vi "update eol result.vi"(7 "Eol数据":string[](array[string]), 11 "Station Index":i32) -> ()   [LabVIEW 2018]
panel:
  in  "error in (no error)":errorcluster
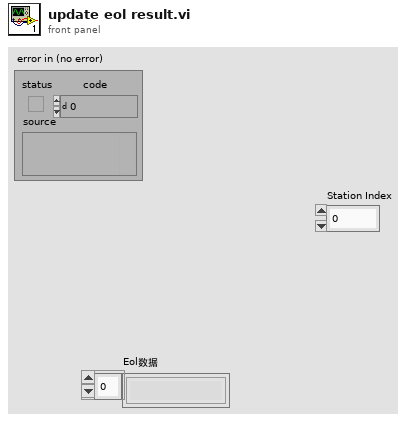
[diagram p1: front panel]
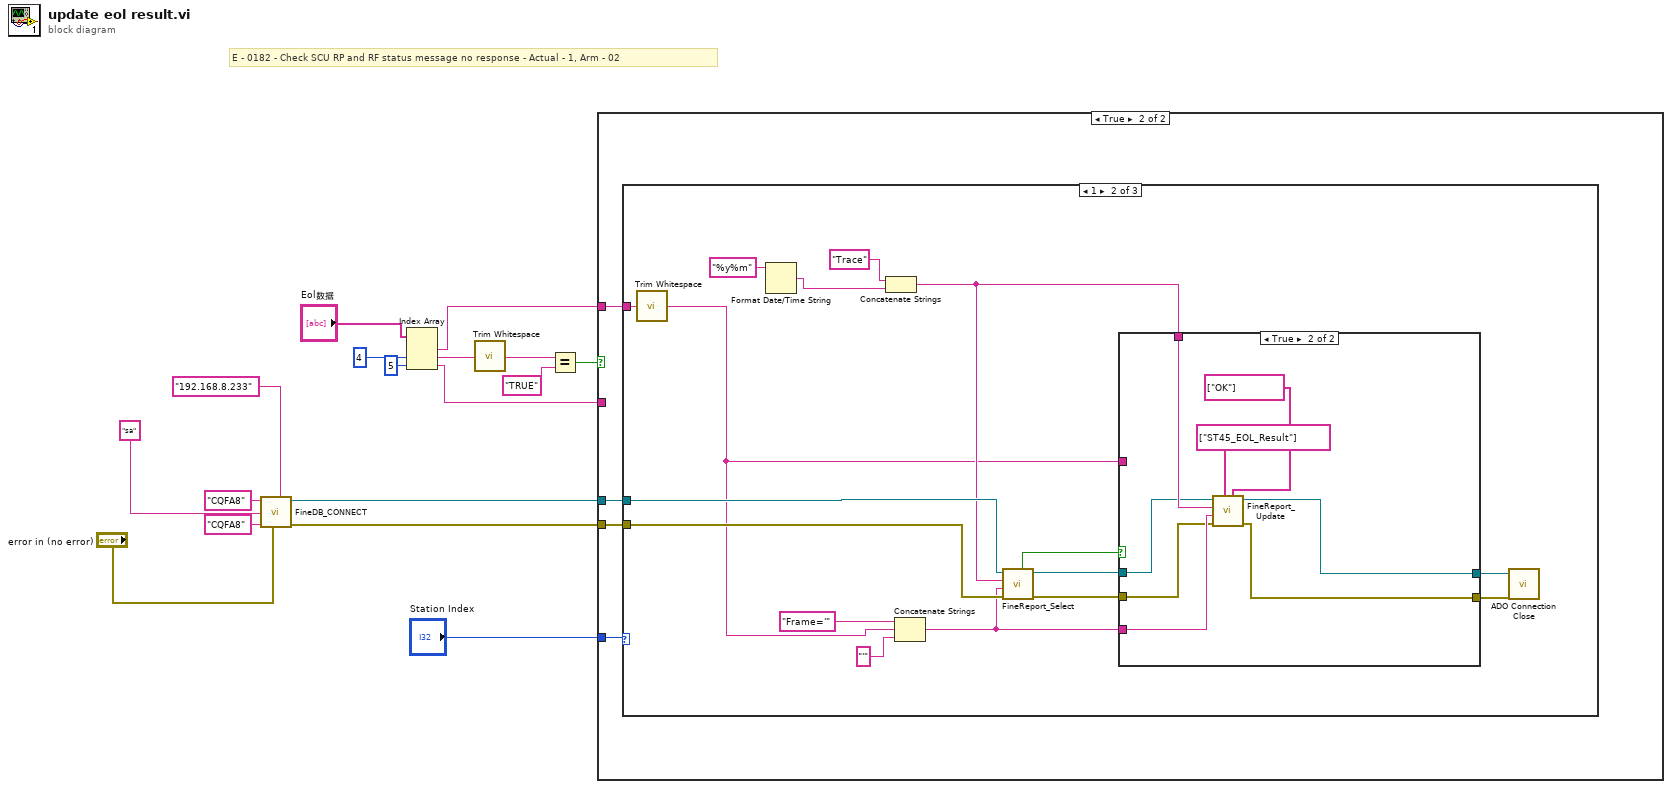
[diagram p0: block diagram]
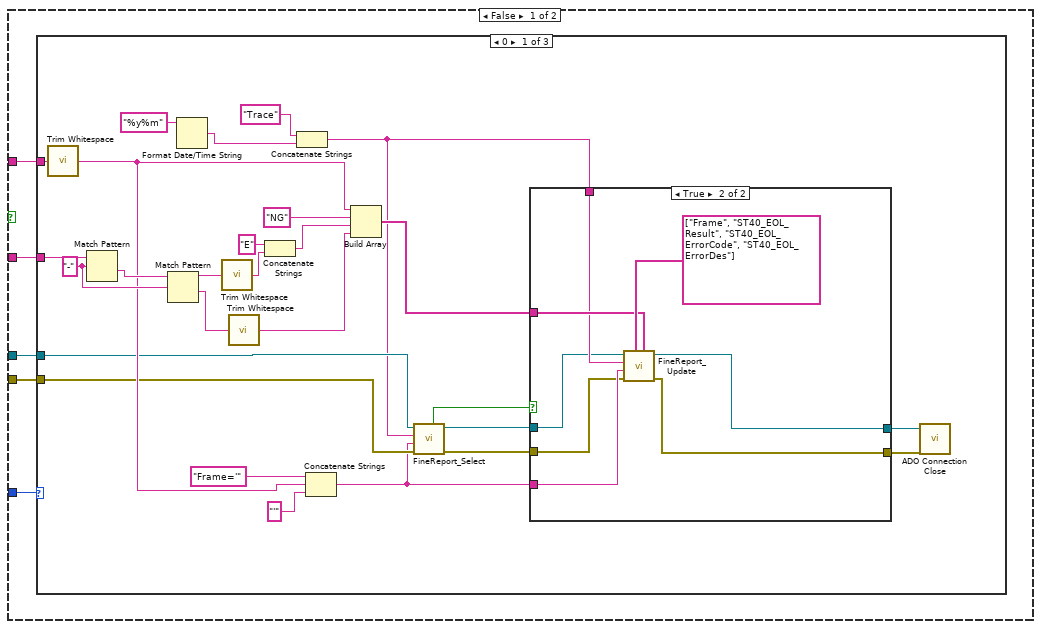
[diagram p2: hidden frame]
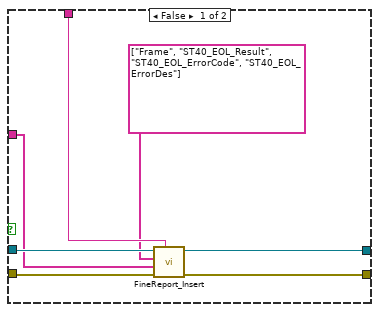
[diagram p3: hidden frame]
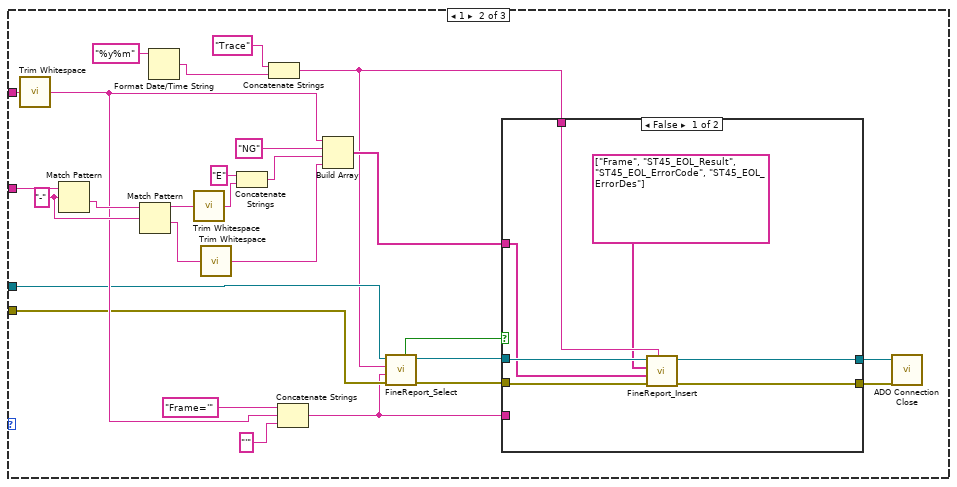
[diagram p4: hidden frame]
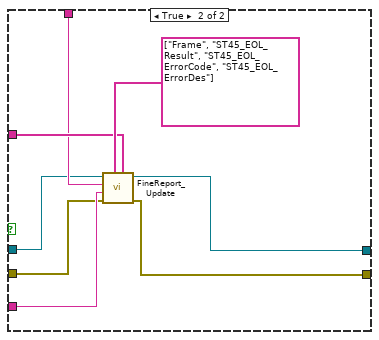
[diagram p5: hidden frame]
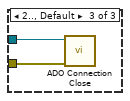
[diagram p6: hidden frame]
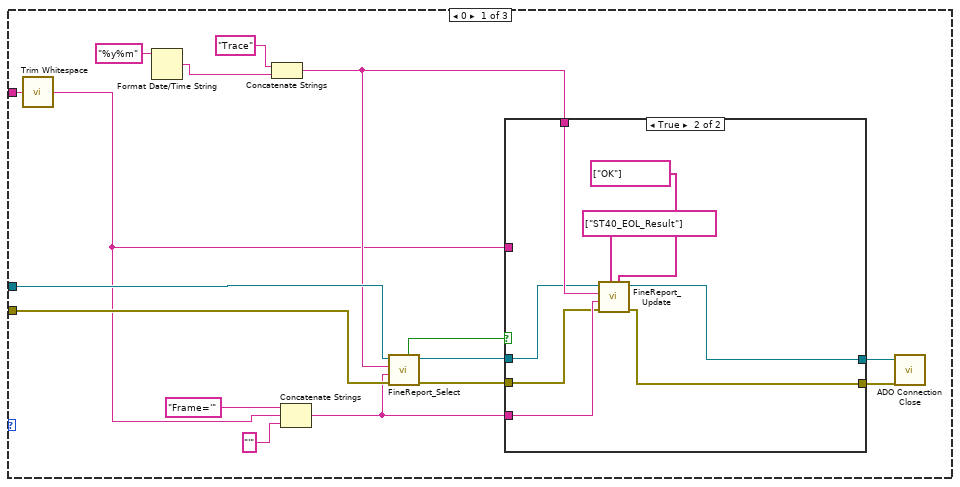
[diagram p7: hidden frame]
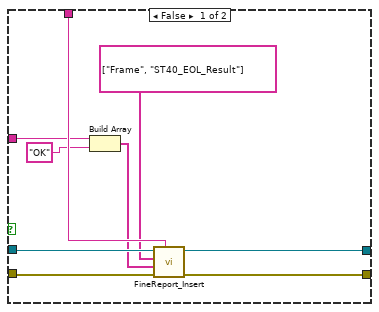
[diagram p8: hidden frame]
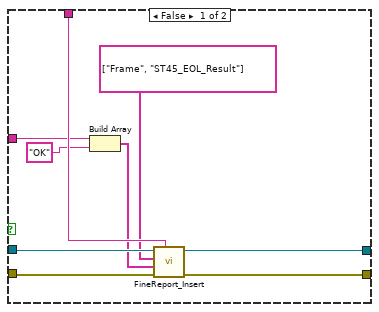
[diagram p9: hidden frame]
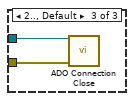
[diagram p10: hidden frame]
diagram:
  # "E - 0182 - Check SCU RP and RF status message no response - Actual - 1, Arm - 02"
  n1 = call "FineDB_CONNECT.vi"("SQL Server_Hostname"="192.168.8.233", "error in (no error)"="error in (no error)", "password"="CQFA8", "account"="sa", "DB_name"="CQFA8") -> ("error out"=w4:errorcluster, "ADODB._Connection Out"=w5:refnum<k7>)  [unwired: 5 in]
  n2 = Index Array(array="Eol数据", index #2=4 ("索引"), index #3=5 ("索引")) -> (element #1=w3:string, element #2=w9:string, element #3=w2:string)  [unwired: 1 in]
  n3 = call <vilib>:"Trim Whitespace.vi"("string"=w9) -> ("trimmed string"=w8:string)  [unwired: 1 in]
  n4 = Equal?(x=w8, y="TRUE") -> (x = y?=w6:bool)
  n5 = case shown="True" w6 {
    tunnel: w5 -> [w20 w111]
    tunnel: w4 -> [w19 w110]
    tunnel: w3 -> [w21 w112]
    tunnel: w2 -> [w22 _]
    tunnel: "Station Index" -> [w18 w109]
    frame False {
      n6 = case shown="0" w18 {
        tunnel: w22 -> [w49 w91 _]
        tunnel: w21 -> [w42 w84 _]
        tunnel: w20 -> [w31 w73 w108]
        tunnel: w19 -> [w30 w72 w107]
        frame 0 {
          w48 = "-" ("正则表达式")
          n7 = call <vilib>:"Trim Whitespace.vi"("string"=w42) -> ("trimmed string"=w34:string)  [unwired: 1 in]
          n8 = Match Pattern(string=w49, regular expression=w48) -> (after substring=w47:string)  [unwired: 1 in, 3 out]
          n9 = Match Pattern(string=w47, regular expression=w48) -> (before substring=w46:string, after substring=w43:string)  [unwired: 1 in, 2 out]
          n10 = Format Date/Time String(time format string (%c)="%y%m" ("时间格式字符串(%c)")) -> (date/time string=w39:string)  [unwired: 2 in]
          n11 = call <vilib>:"Trim Whitespace.vi"("string"=w46) -> ("trimmed string"=w45:string)  [unwired: 1 in]
          n12 = call <vilib>:"Trim Whitespace.vi"("string"=w43) -> ("trimmed string"=w37:string)  [unwired: 1 in]
          n13 = Concatenate Strings("E" ("字符串"), w45) -> (w38:string)
          n14 = Concatenate Strings("Trace", w39) -> (w29:string)
          n15 = Concatenate Strings("Frame='", w34, "'" ("字符串")) -> (w28:string)
          n16 = Build Array(w34, "NG" ("元素"), w38, w37) -> (w32:string[])
          n17 = call "FineReport_Select.vi"("error in (no error)"=w30, "SelectWhere"=w28, "SelectTableName"=w29, "ADODB._Connection in"=w31) -> ("error out"=w25:errorcluster, "ADODB._Connection Out"=w26:refnum<k7>, "有数据"=w27:bool)  [unwired: 3 in, 2 out]
          n18 = case shown="True" w27 {
            tunnel: w32 -> [w52 w63]
            tunnel: w29 -> [w54 w62]
            tunnel: w28 -> [_ w61]
            tunnel: w26 -> [w56 w60]
            tunnel: w25 -> [w55 w59]
            tunnel: [w51 w58] -> w23
            tunnel: [w50 w57] -> w24
            frame False {
              n19 = call "FineReport_Insert.vi"("InsertTableName"=w54, "error in"=w55, "InsertValue(array)"=w52, "InsertColumn(array)"=string[] ["Frame", "ST40_EOL_Result", "ST40_EOL_ErrorCode", "ST40_EOL_ErrorDes"], "ADODB._Connection in"=w56) -> ("error out"=w50:errorcluster, "ADODB._Connection Out"=w51:refnum<k7>)  [unwired: 5 in]
            }
            frame True {
              n20 = call "FineReport_Update.vi"("UpdataValue(array)"=w63, "UpdataColumn(array)"=string[] ["Frame", "ST40_EOL_Result", "ST40_EOL_ErrorCode", "ST40_EOL_ErrorDes"], "error in (no error)"=w59, "UpdataWhere"=w61, "UpdataTableName"=w62, "ADODB._Connection in"=w60) -> ("error out"=w57:errorcluster, "ADODB._Connection Out"=w58:refnum<k7>)  [unwired: 2 in]
            }
          }
          n21 = call <userlib>:"ADO Connection Close.vi"("error in (no error)"=w24, "ADODB._Connection In"=w23) -> ()  [unwired: 8 in, 2 out]
        }
        frame 1 {
          w90 = "-" ("正则表达式")
          n22 = call <vilib>:"Trim Whitespace.vi"("string"=w84) -> ("trimmed string"=w76:string)  [unwired: 1 in]
          n23 = Match Pattern(string=w91, regular expression=w90) -> (after substring=w89:string)  [unwired: 1 in, 3 out]
          n24 = Match Pattern(string=w89, regular expression=w90) -> (before substring=w88:string, after substring=w85:string)  [unwired: 1 in, 2 out]
          n25 = Format Date/Time String(time format string (%c)="%y%m" ("时间格式字符串(%c)")) -> (date/time string=w81:string)  [unwired: 2 in]
          n26 = call <vilib>:"Trim Whitespace.vi"("string"=w88) -> ("trimmed string"=w87:string)  [unwired: 1 in]
          n27 = call <vilib>:"Trim Whitespace.vi"("string"=w85) -> ("trimmed string"=w79:string)  [unwired: 1 in]
          n28 = Concatenate Strings("E" ("字符串"), w87) -> (w80:string)
          n29 = Concatenate Strings("Trace", w81) -> (w71:string)
          n30 = Concatenate Strings("Frame='", w76, "'" ("字符串")) -> (w70:string)
          n31 = Build Array(w76, "NG" ("元素"), w80, w79) -> (w74:string[])
          n32 = call "FineReport_Select.vi"("error in (no error)"=w72, "SelectWhere"=w70, "SelectTableName"=w71, "ADODB._Connection in"=w73) -> ("error out"=w67:errorcluster, "ADODB._Connection Out"=w68:refnum<k7>, "有数据"=w69:bool)  [unwired: 3 in, 2 out]
          n33 = case shown="False" w69 {
            tunnel: w74 -> [w94 w105]
            tunnel: w71 -> [w96 w104]
            tunnel: w70 -> [_ w103]
            tunnel: w68 -> [w98 w102]
            tunnel: w67 -> [w97 w101]
            tunnel: [w93 w100] -> w65
            tunnel: [w92 w99] -> w66
            frame False {
              n34 = call "FineReport_Insert.vi"("InsertTableName"=w96, "error in"=w97, "InsertValue(array)"=w94, "InsertColumn(array)"=string[] ["Frame", "ST45_EOL_Result", "ST45_EOL_ErrorCode", "ST45_EOL_ErrorDes"], "ADODB._Connection in"=w98) -> ("error out"=w92:errorcluster, "ADODB._Connection Out"=w93:refnum<k7>)  [unwired: 5 in]
            }
            frame True {
              n35 = call "FineReport_Update.vi"("UpdataValue(array)"=w105, "UpdataColumn(array)"=string[] ["Frame", "ST45_EOL_Result", "ST45_EOL_ErrorCode", "ST45_EOL_ErrorDes"], "error in (no error)"=w101, "UpdataWhere"=w103, "UpdataTableName"=w104, "ADODB._Connection in"=w102) -> ("error out"=w99:errorcluster, "ADODB._Connection Out"=w100:refnum<k7>)  [unwired: 2 in]
            }
          }
          n36 = call <userlib>:"ADO Connection Close.vi"("error in (no error)"=w66, "ADODB._Connection In"=w65) -> ()  [unwired: 8 in, 2 out]
        }
        frame 2.., Default {
          n37 = call <userlib>:"ADO Connection Close.vi"("error in (no error)"=w107, "ADODB._Connection In"=w108) -> ()  [unwired: 8 in, 2 out]
        }
      }
    }
    frame True {
      n38 = case shown="1" w109 {
        tunnel: w112 -> [w128 w161 _]
        tunnel: w111 -> [w122 w155 w180]
        tunnel: w110 -> [w121 w154 w179]
        frame 0 {
          n39 = call <vilib>:"Trim Whitespace.vi"("string"=w128) -> ("trimmed string"=w113:string)  [unwired: 1 in]
          n40 = Format Date/Time String(time format string (%c)="%y%m" ("时间格式字符串(%c)")) -> (date/time string=w125:string)  [unwired: 2 in]
          n41 = Concatenate Strings("Trace", w125) -> (w120:string)
          n42 = Concatenate Strings("Frame='", w113, "'" ("字符串")) -> (w119:string)
          n43 = call "FineReport_Select.vi"("error in (no error)"=w121, "SelectWhere"=w119, "SelectTableName"=w120, "ADODB._Connection in"=w122) -> ("error out"=w116:errorcluster, "ADODB._Connection Out"=w117:refnum<k7>, "有数据"=w118:bool)  [unwired: 3 in, 2 out]
          n44 = case shown="True" w118 {
            tunnel: w120 -> [w135 w144]
            tunnel: w119 -> [_ w143]
            tunnel: w117 -> [w137 w142]
            tunnel: w116 -> [w136 w141]
            tunnel: [w133 w140] -> w114
            tunnel: [w132 w139] -> w115
            tunnel: w113 -> [w131 _]
            frame False {
              n45 = Build Array(w131, "OK") -> (w129:string[])
              n46 = call "FineReport_Insert.vi"("InsertTableName"=w135, "error in"=w136, "InsertValue(array)"=w129, "InsertColumn(array)"=string[] ["Frame", "ST40_EOL_Result"], "ADODB._Connection in"=w137) -> ("error out"=w132:errorcluster, "ADODB._Connection Out"=w133:refnum<k7>)  [unwired: 5 in]
            }
            frame True {
              n47 = call "FineReport_Update.vi"("UpdataValue(array)"=string[] ["OK"], "UpdataColumn(array)"=string[] ["ST40_EOL_Result"], "error in (no error)"=w141, "UpdataWhere"=w143, "UpdataTableName"=w144, "ADODB._Connection in"=w142) -> ("error out"=w139:errorcluster, "ADODB._Connection Out"=w140:refnum<k7>)  [unwired: 2 in]
            }
          }
          n48 = call <userlib>:"ADO Connection Close.vi"("error in (no error)"=w115, "ADODB._Connection In"=w114) -> ()  [unwired: 8 in, 2 out]
        }
        frame 1 {
          n49 = call <vilib>:"Trim Whitespace.vi"("string"=w161) -> ("trimmed string"=w146:string)  [unwired: 1 in]
          n50 = Format Date/Time String(time format string (%c)="%y%m" ("时间格式字符串(%c)")) -> (date/time string=w158:string)  [unwired: 2 in]
          n51 = Concatenate Strings("Trace", w158) -> (w153:string)
          n52 = Concatenate Strings("Frame='", w146, "'" ("字符串")) -> (w152:string)
          n53 = call "FineReport_Select.vi"("error in (no error)"=w154, "SelectWhere"=w152, "SelectTableName"=w153, "ADODB._Connection in"=w155) -> ("error out"=w149:errorcluster, "ADODB._Connection Out"=w150:refnum<k7>, "有数据"=w151:bool)  [unwired: 3 in, 2 out]
          n54 = case shown="True" w151 {
            tunnel: w153 -> [w168 w177]
            tunnel: w152 -> [_ w176]
            tunnel: w150 -> [w170 w175]
            tunnel: w149 -> [w169 w174]
            tunnel: [w166 w173] -> w147
            tunnel: [w165 w172] -> w148
            tunnel: w146 -> [w164 _]
            frame False {
              n55 = Build Array(w164, "OK") -> (w162:string[])
              n56 = call "FineReport_Insert.vi"("InsertTableName"=w168, "error in"=w169, "InsertValue(array)"=w162, "InsertColumn(array)"=string[] ["Frame", "ST45_EOL_Result"], "ADODB._Connection in"=w170) -> ("error out"=w165:errorcluster, "ADODB._Connection Out"=w166:refnum<k7>)  [unwired: 5 in]
            }
            frame True {
              n57 = call "FineReport_Update.vi"("UpdataValue(array)"=string[] ["OK"], "UpdataColumn(array)"=string[] ["ST45_EOL_Result"], "error in (no error)"=w174, "UpdataWhere"=w176, "UpdataTableName"=w177, "ADODB._Connection in"=w175) -> ("error out"=w172:errorcluster, "ADODB._Connection Out"=w173:refnum<k7>)  [unwired: 2 in]
            }
          }
          n58 = call <userlib>:"ADO Connection Close.vi"("error in (no error)"=w148, "ADODB._Connection In"=w147) -> ()  [unwired: 8 in, 2 out]
        }
        frame 2.., Default {
          n59 = call <userlib>:"ADO Connection Close.vi"("error in (no error)"=w179, "ADODB._Connection In"=w180) -> ()  [unwired: 8 in, 2 out]
        }
      }
    }
  }
